vi "Write Data to LabVIEW INI.vi"(8 "error in":errorcluster, 11 "INI Data":T1={"Show Terminals?"=FALSE, "Text"={"Font"="", "Alignment"=0, "Size"=0}, "3rd party Templates"={"Store 3rd party Templates?"=FALSE, "Folder Name"=""}, "Merge user layers on commit"=FALSE, "Body Text"={"Line 1 text"="", "Line 2 text"="", "Line 3 text"="", "Line 4 text"="", "Line 1 color"=0, "Line 2 color"=0, "Line 3 color"=0, "Line 4 color"=0, "Body Text Spec"={"Font"="", "Alignment"=0, "Size"=3}, "Center text vertically"=FALSE, "Capitalize Text"=FALSE}, "Fill Color"=0, "Edge Color"=0, "Tab"=0, "Tool"=enum."Ellipse", "Disable Layers?"=FALSE} {"Body Text"."Body Text Spec"."Alignment" items=["left", "center", "right"]; "Text"."Alignment" items=["left", "center", "right"]}) -> (0 "error out":errorcluster)   [LabVIEW 2020, in "lv_icon.lvlib"]
uses:
  lv_icon.lvlib
  <resource>/dialog/lvconfig.llb/LV Config Write String.vi
  <resource>/dialog/lvconfig.llb/LV Config Write Color.vi
  <resource>/dialog/lvconfig.llb/LV Config Write Boolean.vi
  vi.lib/LabVIEW Icon API/lv_icon/Controls/IEColor.ctl
  INI Data.ctl
  vi.lib/LabVIEW Icon API/lv_icon/Controls/Font.ctl
  Controls/Circle.ctl
  Controls/Dropper.ctl
  Controls/FCircle.ctl
  Controls/Fill.ctl
  Controls/FRect.ctl
  Controls/Line.ctl
  Controls/Move.ctl
  Controls/Pen.ctl
  Controls/IERect.ctl
  Controls/Rubber.ctl
  Controls/Selection.ctl
  Controls/Text.ctl
  Controls/Tools.ctl
  vi.lib/LabVIEW Icon API/lv_icon/Controls/BodyText.ctl
  Controls/Font Size.ctl
  vi.lib/LabVIEW Icon API/lv_icon/Controls/Alignment.ctl
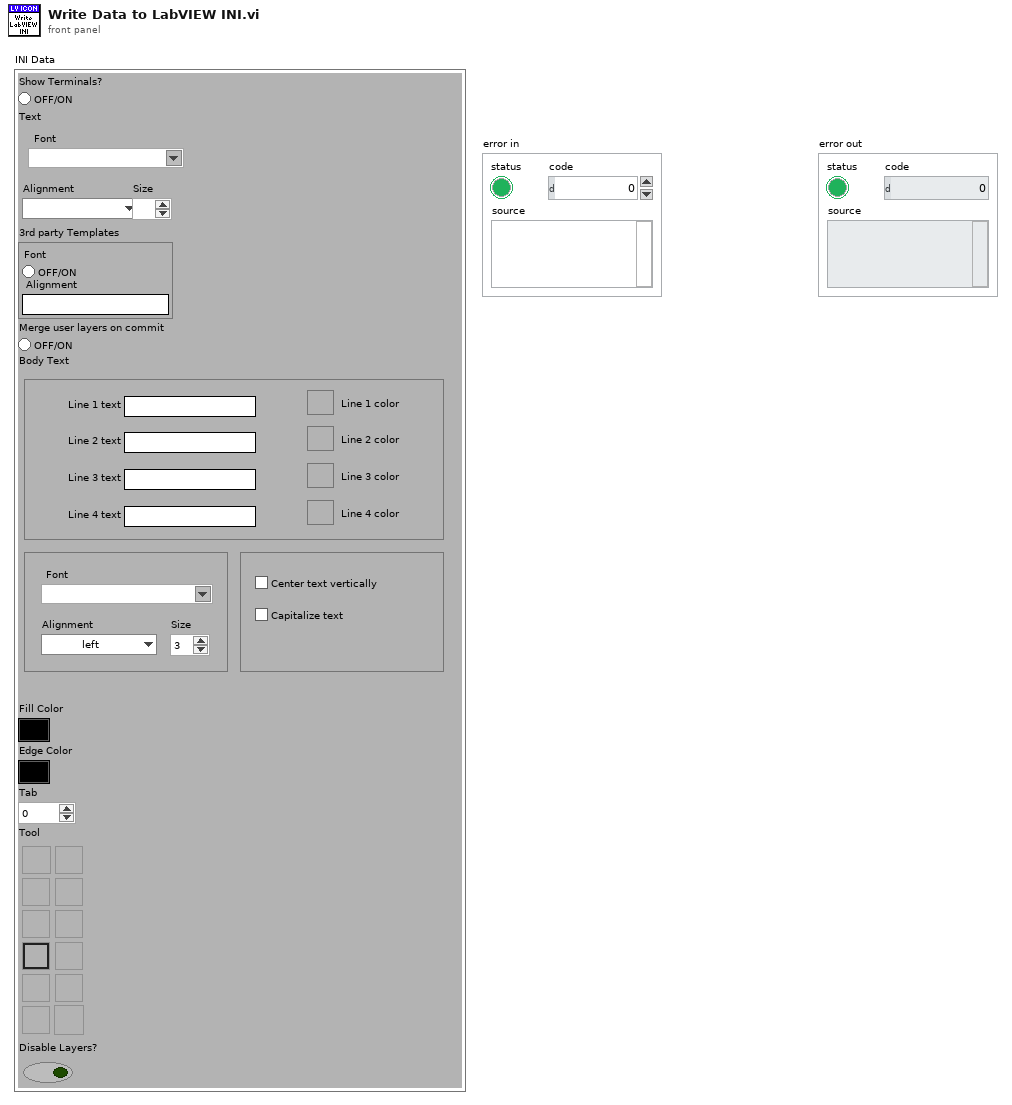
[diagram p1: front panel]
types:
  T1 = typedef "lv_icon.lvlib/INI Data.ctl" = cluster{"Show Terminals?":bool, "Text":cluster{"Font":T2, "Alignment":T3, "Size":T4}, "3rd party Templates":cluster{"Store 3rd party Templates?":bool, "Folder Name":string}, "Merge user layers on commit":bool, "Body Text":T5, "Fill Color":T6, "Edge Color":T6, "Tab":u16, "Tool":T7, "Disable Layers?":bool}
  T2 = typedef "Font.ctl" = string
  T3 = typedef "Alignment.ctl" = u16
  T4 = typedef "Font Size.ctl" = u8
  T5 = typedef "BodyText.ctl" = cluster{"Line 1 text":string, "Line 2 text":string, "Line 3 text":string, "Line 4 text":string, "Line 1 color":u32, "Line 2 color":u32, "Line 3 color":u32, "Line 4 color":u32, "Body Text Spec":cluster{"Font":T2, "Alignment":T3, "Size":u8}, "Center text vertically":bool, "Capitalize Text":bool}
  T6 = typedef "IEColor.ctl" = u32
  T7 = typedef "Tools.ctl" = enum32{"Pencil", "Line", "Dropper", "Fill", "Rectangle", "Filled Rectangle", "Ellipse", "Filled Ellipse", "Eraser", "Text", "Select", "Move"}
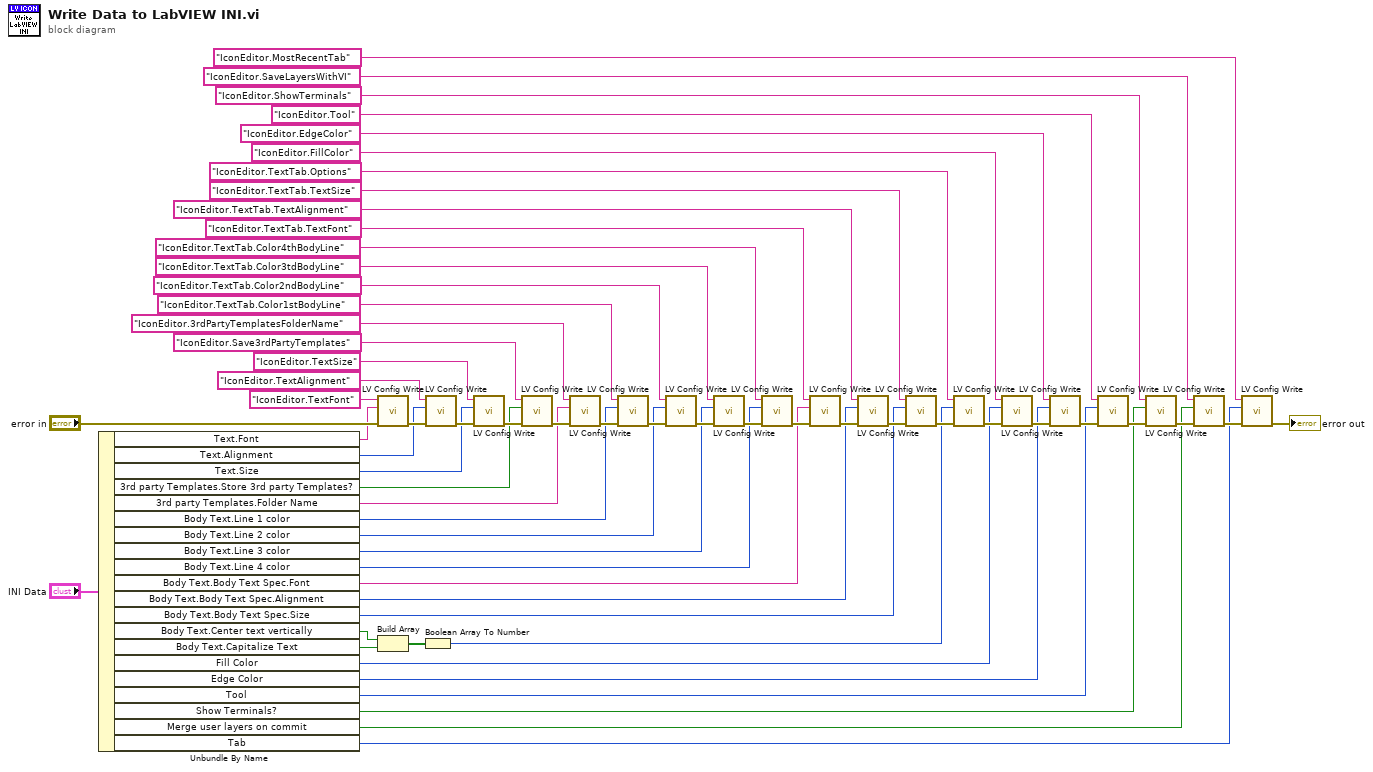
[diagram p0: block diagram]
diagram:
  n1 = Unbundle By Name("INI Data") -> ("Text.Font"=w41:T2, "Text.Alignment"=w39:T3, "Text.Size"=w37:T4, "3rd party Templates.Store 3rd party Templates?"=w35:bool, "3rd party Templates.Folder Name"=w33:string, "Body Text.Line 1 color"=w27:u32, "Body Text.Line 2 color"=w26:u32, "Body Text.Line 3 color"=w25:u32, "Body Text.Line 4 color"=w24:u32, "Body Text.Body Text Spec.Font"=w23:T2, "Body Text.Body Text Spec.Alignment"=w22:T3, "Body Text.Body Text Spec.Size"=w21:u8, "Body Text.Center text vertically"=w16:bool, "Body Text.Capitalize Text"=w17:bool, "Fill Color"=w10:T6, "Edge Color"=w9:T6, "Tool"=w7:T7, "Show Terminals?"=w6:bool, "Merge user layers on commit"=w3:bool, "Tab"=w1:u16)
  n2 = call-poly <resource>:"LV Config Write.vi"("error in (no error)"="error in", "value"=w41, "key"="IconEditor.TextFont") -> ("error out"=w62:errorcluster)  [unwired: 4 out]
  n3 = Build Array(w16, w17) -> (w15:bool[])
  n4 = Boolean Array To Number(Boolean array=w15) -> (number=w13:u32)
  n5 = call-poly <resource>:"LV Config Write.vi"("error in (no error)"=w62, "value"=w39, "key"="IconEditor.TextAlignment") -> ("error out"=w61:errorcluster)  [unwired: 4 in]
  n6 = call-poly <resource>:"LV Config Write.vi"("error in (no error)"=w61, "value"=w37, "key"="IconEditor.TextSize") -> ("error out"=w60:errorcluster)  [unwired: 4 out]
  n7 = call-poly <resource>:"LV Config Write.vi"("error in (no error)"=w60, "value"=w35, "key"="IconEditor.Save3rdPartyTemplates") -> ("error out"=w59:errorcluster)  [unwired: 4 out]
  n8 = call-poly <resource>:"LV Config Write.vi"("error in (no error)"=w59, "value"=w33, "key"="IconEditor.3rdPartyTemplatesFolderName") -> ("error out"=w58:errorcluster)  [unwired: 4 out]
  n9 = call-poly <resource>:"LV Config Write.vi"("error in (no error)"=w58, "value"=w27, "key"="IconEditor.TextTab.Color1stBodyLine") -> ("error out"=w57:errorcluster)  [unwired: 4 out]
  n10 = call-poly <resource>:"LV Config Write.vi"("error in (no error)"=w57, "value"=w26, "key"="IconEditor.TextTab.Color2ndBodyLine") -> ("error out"=w56:errorcluster)  [unwired: 4 out]
  n11 = call-poly <resource>:"LV Config Write.vi"("error in (no error)"=w56, "value"=w25, "key"="IconEditor.TextTab.Color3tdBodyLine") -> ("error out"=w55:errorcluster)  [unwired: 4 out]
  n12 = call-poly <resource>:"LV Config Write.vi"("error in (no error)"=w55, "value"=w24, "key"="IconEditor.TextTab.Color4thBodyLine") -> ("error out"=w54:errorcluster)  [unwired: 4 out]
  n13 = call-poly <resource>:"LV Config Write.vi"("error in (no error)"=w54, "value"=w23, "key"="IconEditor.TextTab.TextFont") -> ("error out"=w53:errorcluster)  [unwired: 4 out]
  n14 = call-poly <resource>:"LV Config Write.vi"("error in (no error)"=w53, "value"=w22, "key"="IconEditor.TextTab.TextAlignment") -> ("error out"=w52:errorcluster)  [unwired: 4 out]
  n15 = call-poly <resource>:"LV Config Write.vi"("error in (no error)"=w52, "value"=w21, "key"="IconEditor.TextTab.TextSize") -> ("error out"=w51:errorcluster)  [unwired: 4 out]
  n16 = call-poly <resource>:"LV Config Write.vi"("error in (no error)"=w51, "value"=w13, "key"="IconEditor.TextTab.Options") -> ("error out"=w50:errorcluster)  [unwired: 4 out]
  n17 = call-poly <resource>:"LV Config Write.vi"("error in (no error)"=w50, "value"=w10, "key"="IconEditor.FillColor") -> ("error out"=w49:errorcluster)  [unwired: 4 out]
  n18 = call-poly <resource>:"LV Config Write.vi"("error in (no error)"=w49, "value"=w9, "key"="IconEditor.EdgeColor") -> ("error out"=w48:errorcluster)  [unwired: 4 out]
  n19 = call-poly <resource>:"LV Config Write.vi"("error in (no error)"=w48, "value"=w7, "key"="IconEditor.Tool") -> ("error out"=w45:errorcluster)  [unwired: 4 out]
  n20 = call-poly <resource>:"LV Config Write.vi"("error in (no error)"=w45, "value"=w6, "key"="IconEditor.ShowTerminals") -> ("error out"=w47:errorcluster)  [unwired: 4 out]
  n21 = call-poly <resource>:"LV Config Write.vi"("error in (no error)"=w47, "value"=w3, "key"="IconEditor.SaveLayersWithVI") -> ("error out"=w46:errorcluster)  [unwired: 4 out]
  n22 = call-poly <resource>:"LV Config Write.vi"("error in (no error)"=w46, "value"=w1, "key"="IconEditor.MostRecentTab") -> ("error out"=→"error out":errorcluster)  [unwired: 4 out]
